vi "set_window_origin.vi"(8 "error_in":errorcluster, 11 "this_vi_reference":refnum<vi>) -> (0 "error_out":errorcluster)   [LabVIEW 2020]
uses:
  <vilib>/Utility/miscctls.llb/LVPointTypeDef.ctl
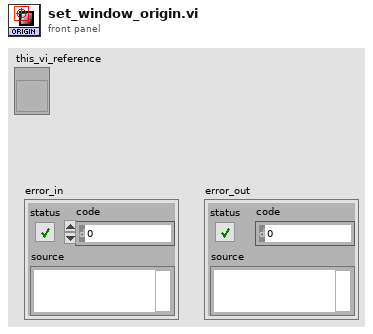
[diagram p1: front panel]
types:
  T1 = typedef "LVPointTypeDef.ctl" = cluster{"Horizontal":i16, "Vertical":i16}
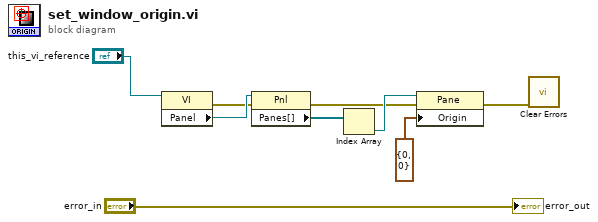
[diagram p0: block diagram]
diagram:
  n1 = property class="VI"(reference="this_vi_reference") -> (error out=w4:errorcluster, "Panel"=w5:refnum<vi>)  [unwired: 1 in, 1 out]
  n2 = property class="Pnl"(reference=w5, error in=w4) -> (error out=w3:errorcluster, "Panes[]"=w6:refnum<vi>[])  [unwired: 1 out]
  n3 = Index Array(array=w6) -> (element=w7:refnum<vi>)  [unwired: 1 in]
  n4 = property class="Pane"(reference=w7, error in=w3, "Origin"=T1 {"Horizontal"=0, "Vertical"=0}) -> (error out=w1:errorcluster)  [unwired: 1 out]
  n5 = call <vilib>:"Clear Errors.vi"("error in (no error)"=w1) -> ()  [unwired: 5 in, 2 out]
  "error_out" <- "error_in"
